vi "Last Ack.vi"(9 "Error":errorcluster, 10 "Actor":refnum<class "Actor.lvclass">, 11 "Last Ack in":refnum<class "Last Ack.lvclass">) -> (0 "error out":errorcluster, 3 "Last Ack out":refnum<class "Last Ack.lvclass">)   [LabVIEW 2021, in "Last Ack.lvlib" / "Last Ack.lvclass"]
uses:
  Last Ack.lvclass
  AAM/Actor/Actor.lvclass
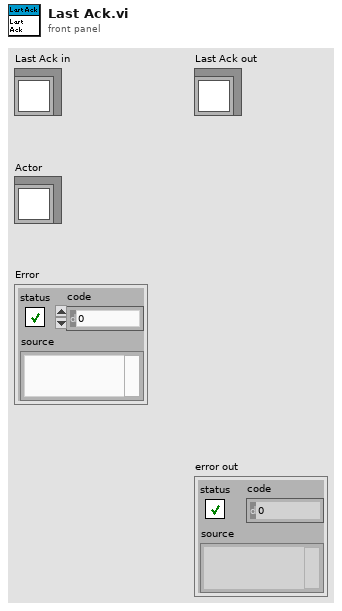
[diagram p1: front panel]
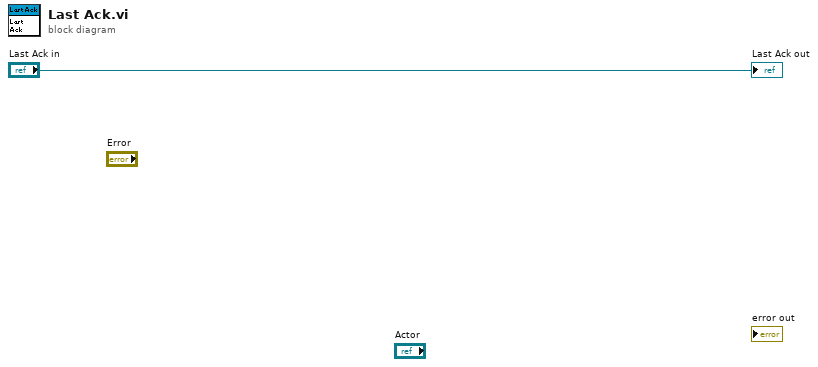
[diagram p0: block diagram]
diagram:
  "Last Ack out" <- "Last Ack in"
